vi "Reserve FGEN Session.vi"(7 "Simulate":bool, 8 "error in (no error)":errorcluster, 9 "Measurement Configuration In":T1={"Start Freq."=100.0, "Freq. Step"=10.0, "Stop Frequ."=1000000.0, "Amplitude"=1.0, "Timing (ms)"=0, "Vin_signal"="Vin_signal", "Vin_measure"="Vin_measure", "Vout_measure"="Vout_measure"} {"Stop Frequ." format="%#_6p"; "Freq. Step" format="%#_6p"; "Start Freq." format="%#_6p"}, 11 "Measurement Context":refnum<class "MeasurementContext.lvclass">) -> (0 "error out":errorcluster, 1 "Measurement Configuration Out":T1={"Start Freq."=100.0, "Freq. Step"=10.0, "Stop Frequ."=1000000.0, "Amplitude"=1.0, "Timing (ms)"=0, "Vin_signal"="Vin_signal", "Vin_measure"="Vin_measure", "Vout_measure"="Vout_measure"} {"Stop Frequ." format="%#_6p"; "Freq. Step" format="%#_6p"; "Start Freq." format="%#_6p"}, 2 "Session":T2, 3 "Measurement Context out":refnum<class "MeasurementContext.lvclass">, 5 "fgen_out":refnum<k15>)   [LabVIEW 2023, in "LabVIEW Bodeplot Summit.lvlib"]
doc: "Reserve Runtime Session for Fgen"
uses:
  LabVIEW Bodeplot Summit.lvlib
  <vilib>/MeasurementLink/MeasurementLink Measurement Server/Classes/MeasurementContext/MeasurementContext.lvclass
  Measurement Configuration.ctl
  Session Info.ctl
  <vilib>/gRPC/LabVIEW gRPC Library/Shared/grpcId.ctl
  <vilib>/MeasurementLink/MeasurementLink Session Management Client/RPC Messages/ni_measurementlink_sessionmanagement_v1_ReserveSessionsResponse.ctl
  <vilib>/MeasurementLink/MeasurementLink Session Management Client/RPC Messages/ni_measurementlink_sessionmanagement_v1_SessionInformation.ctl
  <vilib>/MeasurementLink/MeasurementLink Session Management Client/RPC Messages/nidevice_grpc_Session.ctl
  <vilib>/MeasurementLink/MeasurementLink Session Management Client/RPC Messages/ni_measurementlink_sessionmanagement_v1_ChannelMapping.ctl
  <vilib>/MeasurementLink/MeasurementLink Session Management Client/RPC Messages/ni_measurementlink_sessionmanagement_v1_ReserveSessionsRequest.ctl
  <vilib>/MeasurementLink/MeasurementLink Session Management Client/RPC Messages/ni_measurementlink_PinMapContext.ctl
  <vilib>/MeasurementLink/MeasurementLink Discovery Client/RPC Messages/ni_measurementlink_discovery_v1_ServiceLocation.ctl
  <vilib>/MeasurementLink/MeasurementLink Discovery Client/RPC Messages/ni_measurementlink_discovery_v1_ResolveServiceRequest.ctl
  <instrlib>/niFgen/niFgen.llb/niFgen gRPC Device Server.ctl
  <vilib>/MeasurementLink/MeasurementLink Measurement Server/MeasurementLink Measurement Server.lvlib
  <vilib>/MeasurementLink/MeasurementLink Session Management Client/MeasurementLink Session Management Client.lvlib
  <vilib>/MeasurementLink/MeasurementLink Discovery Client/MeasurementLink Discovery Client.lvlib
  <vilib>/gRPC/LabVIEW gRPC Library/grpc-lvsupport-release.lvlib
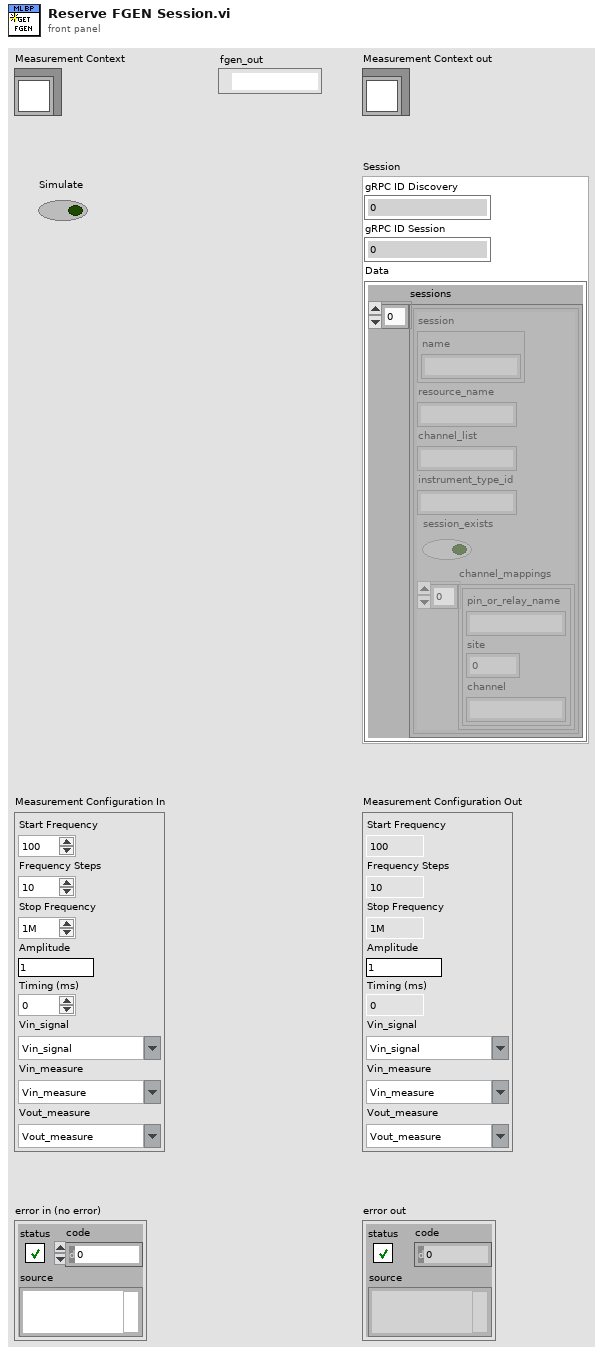
[diagram p1: front panel]
types:
  T1 = typedef "LabVIEW Bodeplot Summit.lvlib/Measurement Configuration.ctl" = cluster{"Start Freq.":dbl, "Freq. Step":dbl, "Stop Frequ.":dbl, "Amplitude":dbl, "Timing (ms)":u32, "Vin_signal":string, "Vin_measure":string, "Vout_measure":string}
  T2 = typedef "LabVIEW Bodeplot Summit.lvlib/Session Info.ctl" = cluster{"gRPC ID Discovery":T3, "gRPC ID Session":T3, "Data":T4}
  T3 = typedef "grpc-lvsupport-release.lvlib/grpcId.ctl" = u64
  T4 = typedef "MeasurementLink Session Management Client.lvlib/ni_measurementlink_sessionmanagement_v1_ReserveSessionsResponse.ctl" = cluster{"sessions":T5[]}
  T5 = typedef "MeasurementLink Session Management Client.lvlib/ni_measurementlink_sessionmanagement_v1_SessionInformation.ctl" = cluster{"session":T6, "resource_name":string, "channel_list":string, "instrument_type_id":string, "session_exists":bool, "channel_mappings":T7[]}
  T6 = typedef "MeasurementLink Session Management Client.lvlib/nidevice_grpc_Session.ctl" = cluster{"name":string}
  T7 = typedef "MeasurementLink Session Management Client.lvlib/ni_measurementlink_sessionmanagement_v1_ChannelMapping.ctl" = cluster{"pin_or_relay_name":string, "site":i32, "channel":string}
  T8 = typedef "MeasurementLink Discovery Client.lvlib/ni_measurementlink_discovery_v1_ServiceLocation.ctl" = cluster{"location":string, "insecure_port":string, "ssl_authenticated_port":string}
  T9 = typedef "MeasurementLink Session Management Client.lvlib/ni_measurementlink_sessionmanagement_v1_ReserveSessionsRequest.ctl" = cluster{"pin_map_context":T10, "pin_or_relay_names":string[], "instrument_type_id":string, "timeout_in_milliseconds":i32}
  T10 = typedef "MeasurementLink Session Management Client.lvlib/ni_measurementlink_PinMapContext.ctl" = cluster{"pin_map_id":string, "sites":i32[]}
  T11 = typedef "MeasurementLink Measurement Server.lvlib/PinMapContext.ctl" = cluster{"pin_map_id":string, "sites":i32[]}
  T12 = typedef "MeasurementLink Discovery Client.lvlib/ni_measurementlink_discovery_v1_ResolveServiceRequest.ctl" = cluster{"provided_interface":string, "service_class":string}
  T13 = typedef "niFgen gRPC Device Server.ctl" = cluster{"Session Name":string, "Address (localhost)":string, "Port (31763)":u32}
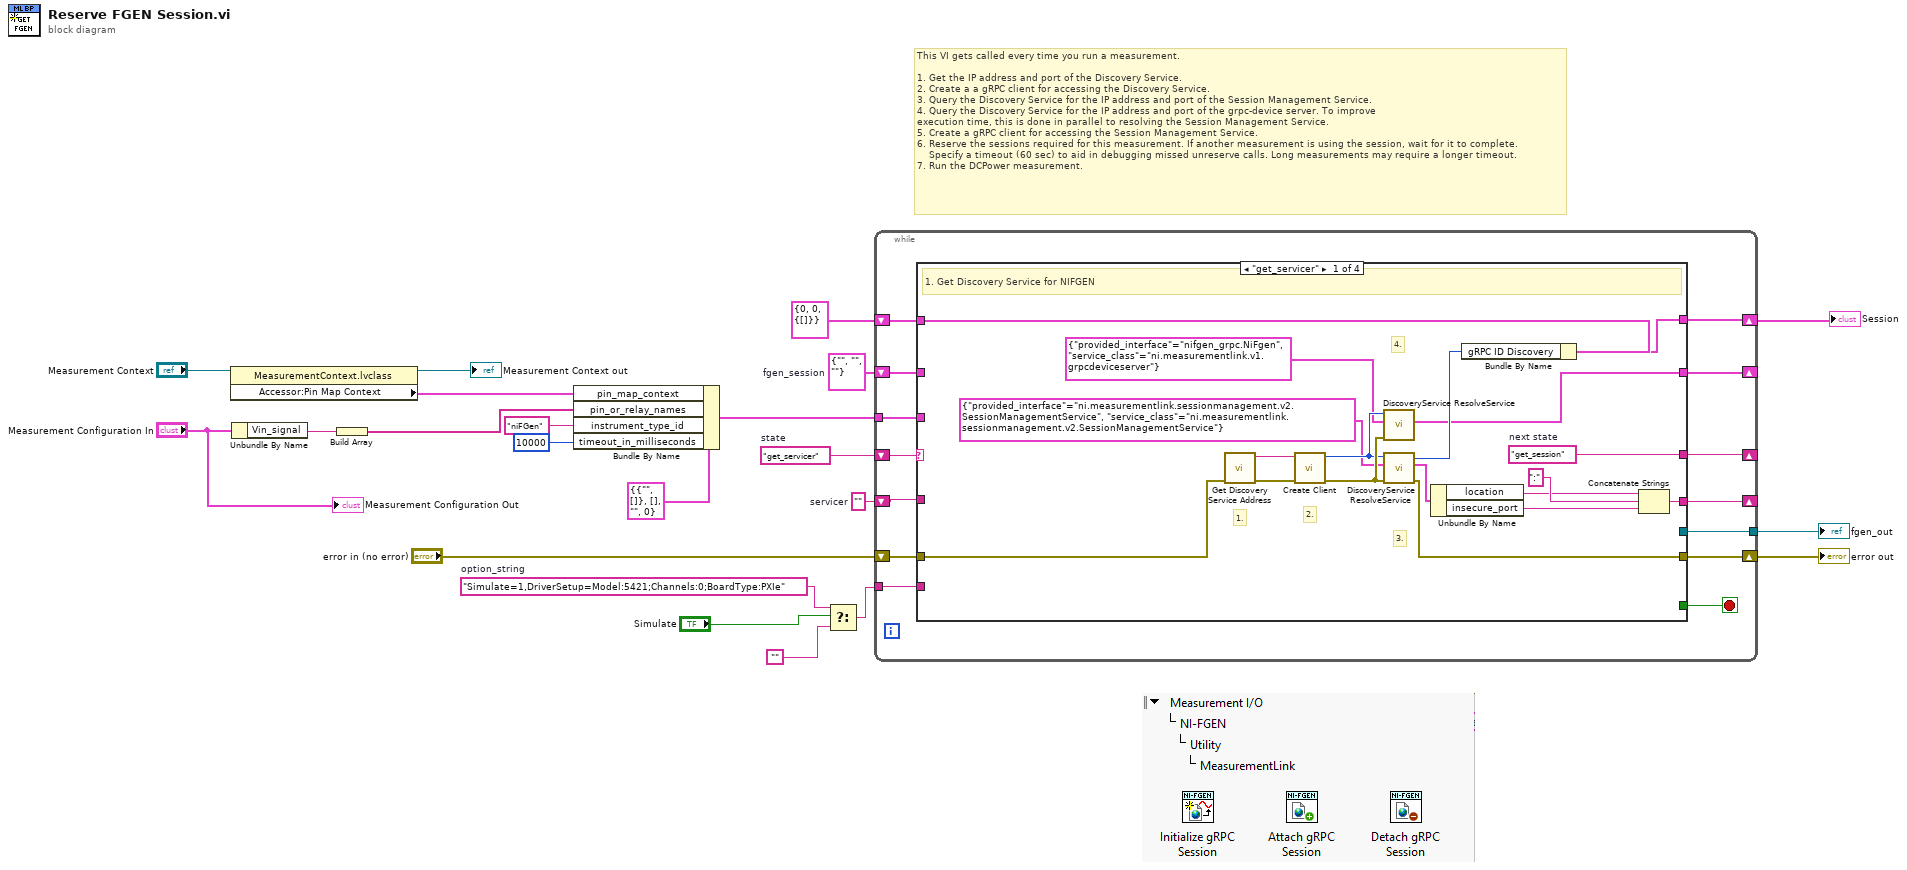
[diagram p0: block diagram]
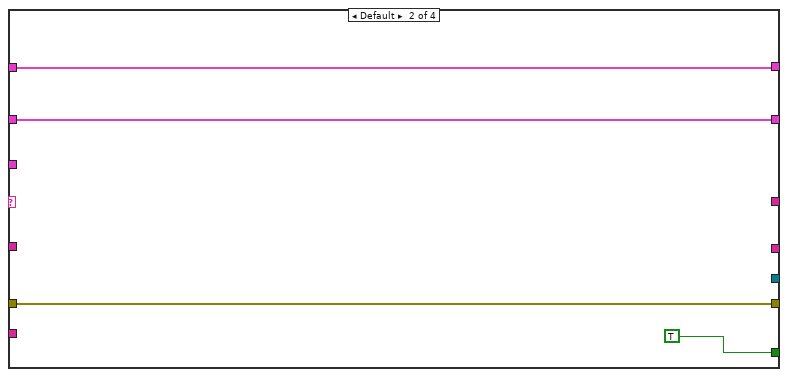
[diagram p2: hidden frame]
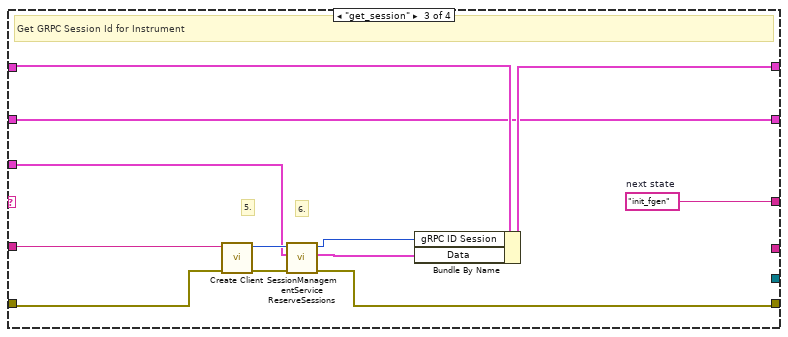
[diagram p3: hidden frame]
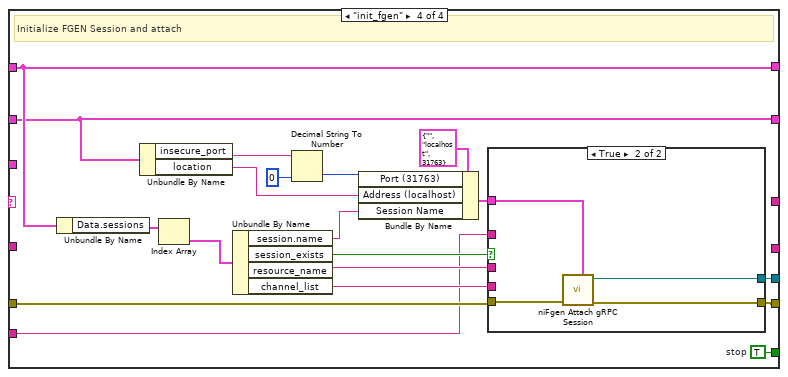
[diagram p4: hidden frame]
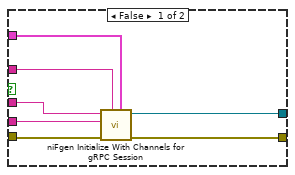
[diagram p5: hidden frame]
diagram:
  w8 = T8 {"location"="", "insecure_port"="", "ssl_authenticated_port"=""}  # fgen_session
  w11 = ""  # servicer
  w14 = "get_servicer"  # state
  w3 = "Simulate=1,DriverSetup=Model:5421;Channels:0;BoardType:PXIe"  # option_string
  # "This VI gets called every time you run a measurement.\n\n1. Get the IP address and port of the Discovery Service.\n2. Create a a gRPC client for accessing the Discovery Service.\n3. Query the Discovery Service for the IP address and port of the Session Management Service.\n4. Query the Discovery Service for the IP address and port of the grpc-device server. To improve \nexecution time, this is done in parallel to resolving the Session Management Service.\n5. Create a gRPC client for accessing the Session Management Service.\n6. Reserve the sessions required for this measurement. If another measurement is using the session, wait for it to complete. \n    Specify a timeout (60 sec) to aid in debugging missed unreserve calls. Long measurements may require a longer timeout.\n7. Run the DCPower measurement."
  n1 = property class="MeasurementContext.lvclass"(reference="Measurement Context") -> (reference out=→"Measurement Context out":refnum<class "MeasurementContext.lvclass">, "Accessor:Pin Map Context"=w20:T11)  [unwired: 1 in, 1 out]
  n2 = Unbundle By Name("Measurement Configuration In") -> ("Vin_signal"=w16:string)
  n3 = Build Array(w16) -> (w15:string[])
  n4 = Bundle By Name(cluster=T9 {"pin_map_context"={"pin_map_id"="", "sites"=[]}, "pin_or_relay_names"=[], "instrument_type_id"="", "timeout_in_milliseconds"=0} ("Request Data"), "pin_map_context"=w20, "pin_or_relay_names"=w15, "instrument_type_id"="niFGen" ("Instrument Type Id"), "timeout_in_milliseconds"=10000) -> (w10:T9)
  n5 = Select(t=w3, s="Simulate", f="") -> (s? t:f=w2:string)
  n6 = while {
    shift-right: [w30] -> _
    shift-left: w14 -> [w36]
    shift-right: [w32] -> w9
    shift-left: T2 {"gRPC ID Discovery"=0, "gRPC ID Session"=0, "Data"={"sessions"=[]}} ("Session") -> [w33]
    shift-right: [w31] -> _
    shift-left: w11 -> [w29]
    shift-right: [w34] -> w6
    shift-left: "error in (no error)" -> [w35]
    tunnel: w10 -> [w28]
    shift-right: [w27] -> _
    shift-left: w8 -> [w26]
    tunnel: w2 -> [w25]
    tunnel: [w24] -> w7
    stop <- w23 stop-if-true
    n7 = case shown="\"get_servicer\"" w36 {
      tunnel: w35 -> [w48 w56 w67 w75]
      tunnel: [w47 w56 w62 w74] -> w34
      tunnel: w33 -> [w46 w58 w65 w88]
      tunnel: [w45 w58 w63 w88] -> w32
      tunnel: [w39 _ _ _] -> w31
      tunnel: [w38 _ w60 _] -> w30
      tunnel: w29 -> [_ _ w68 _]
      tunnel: w28 -> [_ _ w66 _]
      tunnel: [w37 w57 w59 w76] -> w27
      tunnel: w26 -> [_ w57 w59 w76]
      tunnel: w25 -> [_ _ _ w71]
      tunnel: [_ _ _ w73] -> w24
      tunnel: [_ TRUE _ w72] -> w23
      frame "get_servicer" {
        w38 = "get_session"  # next state
        # "4."
        # "3."
        # "2."
        # "1."
        # "1. Get Discovery Service for NIFGEN"
        n8 = call <vilib>:"Get Discovery Service Address.vi"("error in"=w48) -> ("error out"=w51:errorcluster, "address"=w52:string)  [unwired: 9 in]
        n9 = call <vilib>:"Create Client.vi"("error in"=w51, "address"=w52) -> ("error out"=w54:errorcluster, "gRPC ID Out"=w53:T3)  [unwired: 8 in]
        n10 = call <vilib>:"DiscoveryService ResolveService.vi"("error in"=w54, "Request Data"=T12 {"provided_interface"="nifgen_grpc.NiFgen", "service_class"="ni.measurementlink.v1.grpcdeviceserver"}, "gRPC ID"=w53) -> ("Response Data"=w37:T8)  [unwired: 6 in, 2 out]
        n11 = call <vilib>:"DiscoveryService ResolveService.vi"("error in"=w54, "Request Data"=T12 {"provided_interface"="ni.measurementlink.sessionmanagement.v2.SessionManagementService", "service_class"="ni.measurementlink.sessionmanagement.v2.SessionManagementService"}, "gRPC ID"=w53) -> ("error out"=w47:errorcluster, "Response Data"=w42:T8, "gRPC ID out"=w44:T3)  [unwired: 6 in]
        n12 = Unbundle By Name(w42) -> ("location"=w41:string, "insecure_port"=w40:string)
        n13 = Bundle By Name(cluster=w46, "gRPC ID Discovery"=w44) -> (w45:T2)
        n14 = Concatenate Strings(w41, ":" ("string"), w40) -> (w39:string)
      }
      frame Default {
      }
      frame "get_session" {
        w60 = "init_fgen"  # next state
        # "6."
        # "5."
        # "Get GRPC Session Id for Instrument"
        n15 = call <vilib>:"Create Client.vi"("error in"=w67, "address"=w68) -> ("error out"=w70:errorcluster, "gRPC ID Out"=w69:T3)  [unwired: 8 in]
        n16 = call <vilib>:"SessionManagementService ReserveSessions.vi"("error in"=w70, "Request Data"=w66, "gRPC ID"=w69) -> ("error out"=w62:errorcluster, "Response Data"=w64:T4, "gRPC ID out"=w61:T3)  [unwired: 6 in]
        n17 = Bundle By Name(cluster=w65, "gRPC ID Session"=w61, "Data"=w64) -> (w63:T2)
      }
      frame "init_fgen" {
        w72 = TRUE  # stop
        # "Initialize FGEN Session and attach"
        n18 = Unbundle By Name(w88) -> ("Data.sessions"=w89:T5[])
        n19 = Unbundle By Name(w76) -> ("insecure_port"=w84:string, "location"=w83:string)
        n20 = Index Array(array=w89) -> (element=w77:T5)  [unwired: 1 in]
        n21 = Unbundle By Name(w77) -> ("session.name"=w82:string, "session_exists"=w80:bool, "resource_name"=w86:string, "channel_list"=w87:string)
        n22 = Decimal String To Number(string=w84, default (0L)=u32 0 ("Port (31763)")) -> (number=w85:u32)  [unwired: 1 in, 1 out]
        n23 = Bundle By Name(cluster=T13 {"Session Name"="", "Address (localhost)"="localhost", "Port (31763)"=31763} ("gRPC Options"), "Port (31763)"=w85, "Address (localhost)"=w83, "Session Name"=w82) -> (w81:T13)
        n24 = case shown="True" w80 {
          tunnel: w75 -> [w91 w100]
          tunnel: w81 -> [w95 w99]
          tunnel: [w94 w98] -> w74
          tunnel: [w96 w97] -> w73
          tunnel: w86 -> [w93 _]
          tunnel: w87 -> [w92 _]
          tunnel: w71 -> [w90 _]
          frame False {
            n25 = call <instrlib>:"niFgen Initialize With Channels for gRPC Session.vi"("gRPC Options"=w95, "Option String"=w90, "error in (no error)"=w91, "Channel Name"=w92, "Resource Name"=w93) -> ("error out"=w94:errorcluster, "Instrument Handle Out"=w96:refnum<k15>)  [unwired: 5 in]
          }
          frame True {
            n26 = call <instrlib>:"niFgen Attach gRPC Session.vi"("gRPC Options"=w99, "error in (no error)"=w100) -> ("error out"=w98:errorcluster, "Instrument Handle Out"=w97:refnum<k15>)  [unwired: 8 in]
          }
        }
      }
    }
  }
  "error out" <- w6
  "fgen_out" <- w7
  "Session" <- w9
  "Measurement Configuration Out" <- "Measurement Configuration In"
